vi "replace_sub_array (SubVI).vi"(0 "Array in":dbl[][](array[numeric]), 1 "replace arr":dbl[](array[numeric]), 2 "row":i32, 3 "start col":i32) -> (6 "Array out":dbl[][](array[numeric]))   [LabVIEW 2014]
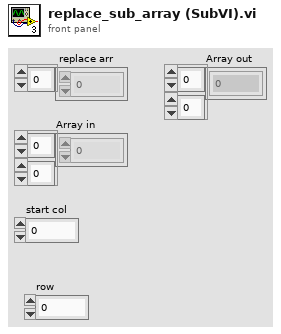
[diagram p1: front panel]
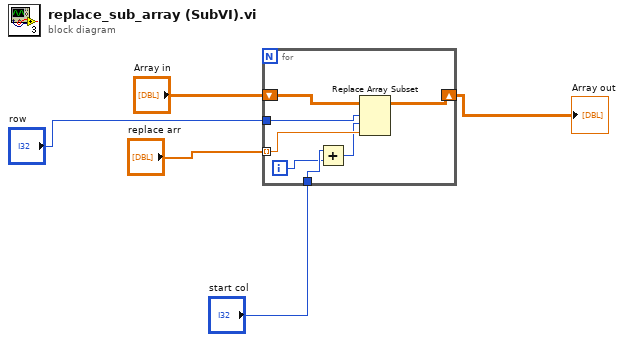
[diagram p0: block diagram]
diagram:
  n1 = for {
    tunnel: "start col" -> [w8]
    shift-right: [w11] -> w1
    shift-left: "Array in" -> [w12]
    tunnel: "replace arr" -> [w10] mode=indexing
    tunnel: "row" -> [w9]
    i -> [w7]
    n2 = Add(x=w8, y=w7) -> (x+y=w6:i32)
    n3 = Replace Array Subset(array=w12, new element=w10, index (row)=w9, index (col)=w6) -> (w11:dbl[][])
  }
  "Array out" <- w1
